vi "Parallel Process Markov Chains.vi"(6 "Suggestion Limit":u16=4, 7 "Queue in":refnum<queue>, 8 "error in (no error)":errorcluster, 9 "Parallel Instances (8)":i32=8, 10 "Progress ref in":refnum<vi>, 11 "Pattern Frequencies":map{string[], i32}(c390)) -> (0 "error out":errorcluster, 3 "Map":T1(c390))   [LabVIEW 2024]
uses:
  Indexer Action.ctl
  <vilib>/Utility/miscctls.llb/LVMapReplaceAction.ctl
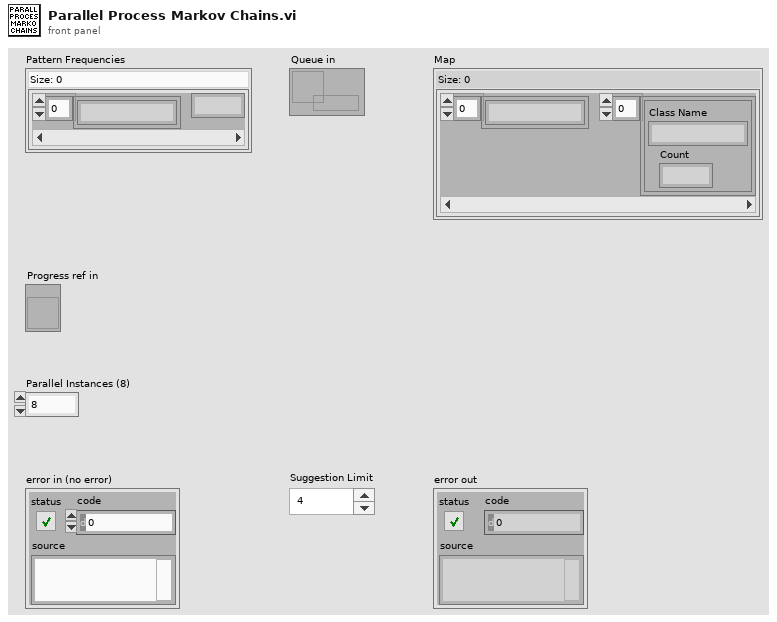
[diagram p1: front panel]
types:
  T1 = map{string[], cluster{"Class Name":string, "Count":i32}[]}
  T2 = map{string[], cluster{"Count":i32, "Class Name":string}[]}
  T3 = typedef "LVMapReplaceAction.ctl" = enum32{"Modify Entry only if found", "Add or Modify Entry", "Delete Entry"}
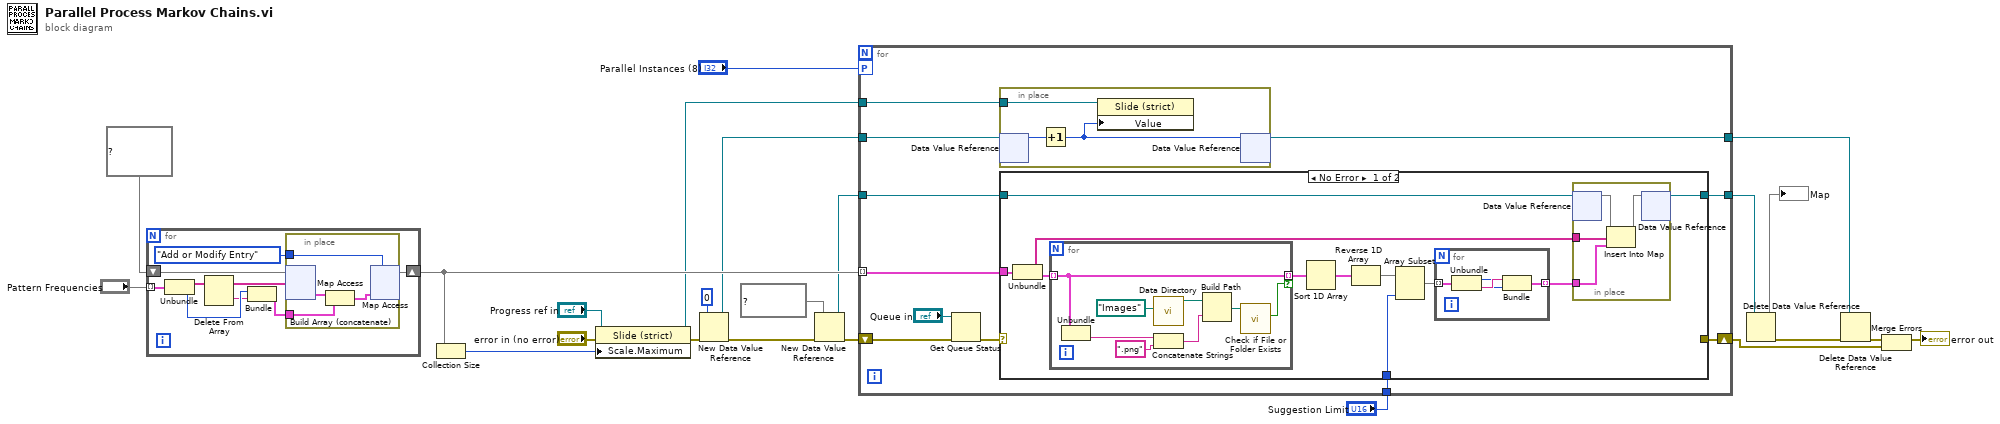
[diagram p0: block diagram]
diagram:
  n1 = for {
    tunnel: "Pattern Frequencies" -> [w32] mode=indexing
    shift-right: [w27] -> w22
    shift-left: T2 {} ("Map") -> [w28]
    n2 = Unbundle(w32) -> (w31:string[], w26:i32)
    n3 = Delete From Array(array=w31) -> (deleted portion=w25:string, array with subset deleted=w30:string[])  [unwired: 2 in]
    n4 = Bundle(w26, "Class Name"=w25) -> (w29:cluster{i32, "Class Name":string})  [unwired: 1 in]
    n5 = in-place {
      in-place-border: w29 -> [w35]
      in-place-border: LVMapReplaceAction."Add or Modify Entry" ("action") -> [w33]
      n6 = in-place-map #1(w28, w30) -> (w36:cluster{"Count":i32, "Class Name":string}[])  [unwired: 1 in, 1 out]
      n7 = Build Array (concatenate)(w36, w35) -> (w34:cluster{"Count":i32, "Class Name":string}[])
      n8 = in-place-map #1(w34, w33) -> (w27:T2)  [unwired: 2 out]
    }
  }
  n9 = Collection Size(1:w22) -> (0:w14:i32)
  n10 = property on="Property Node" class="Slide (strict)"(reference="Progress ref in", error in="error in (no error)", "Scale.Maximum"=w14) -> (reference out=w12:refnum<vi>, error out=w15:errorcluster)
  n11 = New Data Value Reference(data value=u64 0, error in=w15) -> (data value reference=w20:refnum<data-value>, error out=w9:errorcluster)
  n12 = New Data Value Reference(data value=T1 {} ("Map"), error in=w9) -> (data value reference=w8:refnum<data-value>, error out=w10:errorcluster)
  n13 = for {
    tunnel: w22 -> [w47] mode=indexing
    tunnel: "Suggestion Limit" -> [w46]
    shift-right: [w43] -> w2
    shift-left: w10 -> [w44]
    workers-P: "Parallel Instances (8)" -> [_]
    tunnel: w20 -> [w42]
    tunnel: [w41] -> w19
    tunnel: w12 -> [w39]
    tunnel: w8 -> [w38]
    tunnel: [w37] -> w5
    n14 = Get Queue Status(queue="Queue in", error in (no error)=w44) -> (error out=w45:errorcluster)  [unwired: 1 in, 7 out]
    n15 = in-place {
      in-place-border: w39 -> [w49]
      n16 = in-place-dvr #2(w42) -> (w50:u64)  [unwired: 1 out]
      n17 = Increment(x=w50) -> (x+1=w48:u64)
      n18 = property class="Slide (strict)"(reference=w49, "Value"=w48) -> ()  [unwired: 1 in, 2 out]
      n19 = in-place-dvr #2(w48) -> (w41:refnum<data-value>)  [unwired: 1 out]
    }
    n20 = case shown="No Error" w45 {
      selector: w45 -> [_ w79]
      tunnel: w47 -> [w61 _]
      tunnel: w46 -> [w55 _]
      tunnel: [_ w79] -> w43
      tunnel: w38 -> [w54 w78]
      tunnel: [w51 w78] -> w37
      frame No Error {
        n21 = Unbundle(w61) -> (w53:string[], w57:cluster{"Count":i32, "Class Name":string}[])
        n22 = for {
          tunnel: w57 -> [w73] mode=indexing
          tunnel: [w73] -> w56 mode=indexing if=w68
          n23 = Unbundle(w73) -> ("Class Name"=w69:string)  [unwired: 1 out]
          n24 = call "Data Directory.vi"("Subdirectory"=path "Images" ("name or relative path")) -> ("Data directory"=w66:path)  [unwired: 9 in, 1 out]
          n25 = Concatenate Strings(w69, ".png" ("string")) -> (w71:string)
          n26 = Build Path(base path=w66, name or relative path=w71) -> (appended path=w72:path)
          n27 = call <vilib>:"Check if File or Folder Exists.vi"("path"=w72) -> ("file or folder exists?"=w68:bool)  [unwired: 8 in, 2 out]
        }
        n28 = Sort 1D Array(array=w56) -> (sorted array=w59:cluster{"Count":i32, "Class Name":string}[])
        n29 = Reverse 1D Array(array=w59) -> (reversed array=w58:cluster{"Count":i32, "Class Name":string}[])
        n30 = Array Subset(array=w58, length=w55) -> (w60:cluster{"Count":i32, "Class Name":string}[])  [unwired: 1 in]
        n31 = for {
          tunnel: w60 -> [w77] mode=indexing
          tunnel: [w76] -> w52 mode=indexing
          n32 = Unbundle(w77) -> ("Count"=w74:i32, "Class Name"=w75:string)
          n33 = Bundle("Class Name"=w75, "Count"=w74) -> (w76:cluster{"Class Name":string, "Count":i32})  [unwired: 1 in]
        }
        n34 = in-place {
          in-place-border: w53 -> [w63]
          in-place-border: w52 -> [w62]
          n35 = in-place-dvr #3(w54) -> (w65:T1)  [unwired: 1 out]
          n36 = Insert Into Map(map in=w65, key=w63, value=w62) -> (map out=w64:T1)  [unwired: 2 out]
          n37 = in-place-dvr #3(w64) -> (w51:refnum<data-value>)  [unwired: 1 out]
        }
      }
      frame Error {
      }
    }
  }
  n38 = Delete Data Value Reference(data value reference=w5) -> (data value=→"Map":T1, error out=w6:errorcluster)  [unwired: 1 in]
  n39 = Delete Data Value Reference(data value reference=w19, error in=w6) -> (error out=w3:errorcluster)  [unwired: 1 out]
  n40 = Merge Errors(w3, w2) -> (→"error out":errorcluster)
